vi "Save JSON File.vi"(8 "error in (no error)":errorcluster, 10 "Data":variant, 11 "Control Experiment in":refnum<class "Control Experiment.lvclass">) -> (0 "error out":errorcluster)   [LabVIEW 2016, in "Control Experiment.lvclass"]
uses:
  Control Experiment.lvclass
  Control Experiment.lvclass/Control Experiment.ctl
  <vilib>/addons/_JKI.lib/Serialization/JSON/JKI JSON Serialization.lvlib
panel:
  out "Control Experiment out":refnum<class "Control Experiment.lvclass">
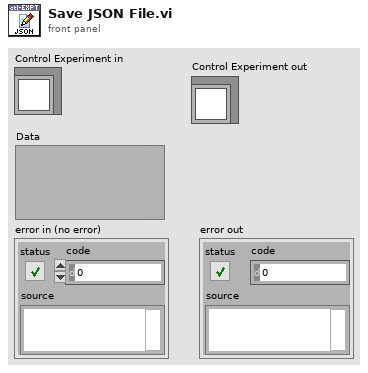
[diagram p1: front panel]
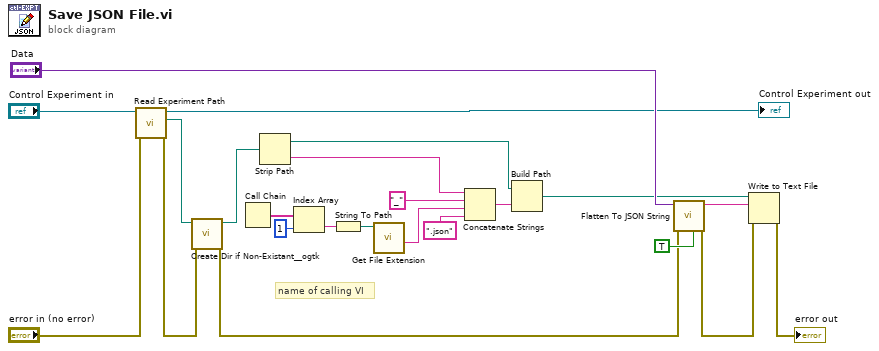
[diagram p0: block diagram]
diagram:
  # "name of calling VI"
  n1 = call "Read Experiment Path.vi"("error in (no error)"="error in (no error)", "Control Experiment in"="Control Experiment in") -> ("error out"=w13:errorcluster, "Experiment Path"=w4:path, "Control Experiment out"=→"Control Experiment out":refnum<class "Control Experiment.lvclass">)  [unwired: 7 in]
  n2 = call <userlib>:"Create Dir if Non-Existant__ogtk.vi"("error in (no error)"=w13, "Directory Path"=w4) -> ("error out"=w12:errorcluster, "dup Directory Path"=w3:path)  [unwired: 7 in, 1 out]
  n3 = Call Chain() -> (call chain=w19:string[])
  n4 = Strip Path(path=w3) -> (stripped path=w6:path, name=w5:string)
  n5 = Index Array(array=w19, index=1) -> (element=w20:string)
  n6 = String To Path(string=w20) -> (path=w22:path)
  n7 = call <vilib>:"Get File Extension.vi"("file"=w22) -> ("filename without extension"=w8:string)  [unwired: 6 in, 4 out]
  n8 = Concatenate Strings(w5, "_" ("string"), w8, ".json" ("string")) -> (w17:string)
  n9 = Build Path(base path=w6, name or relative path=w17) -> (appended path=w2:path)
  n10 = call <vilib>:"Flatten To JSON String.vi"("Enums As String (F)"=TRUE, "error in (no error)"=w12, "Variant"="Data") -> ("error out"=w11:errorcluster, "JSON String"=w16:string)  [unwired: 7 in]
  n11 = Write to Text File(file (use dialog)=w2, text=w16, error in=w11) -> (error out=→"error out":errorcluster)  [unwired: 1 in, 2 out]
